vi "PDF Pfad Warnung.vi"(10 "Sprachliste":string[][](array[string]), 11 "String":string) -> ()   [LabVIEW 2015, in "Linearisierung.lvlib"]
uses:
  Linearisierung/Linearisierung.lvlib
  Sprachverwaltung/Sprachverwaltung.lvlib
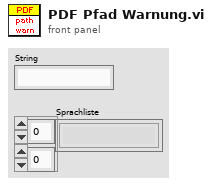
[diagram p1: front panel]
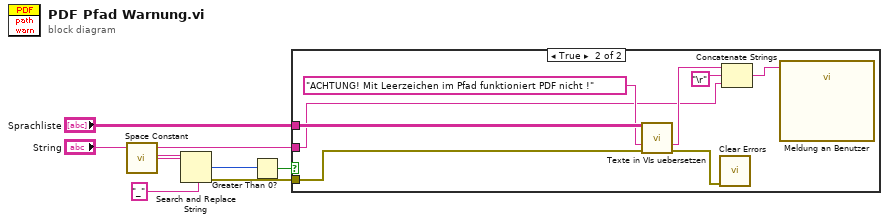
[diagram p0: block diagram]
diagram:
  n1 = call <vilib>:"Space Constant.vi"() -> ("String"=w2:string)
  n2 = Search and Replace String(input string="String", search string=w2, replace string="_") -> (number of replacements=w4:i32, error out=w7:errorcluster)  [unwired: 5 in, 2 out]
  n3 = Greater Than 0?(x=w4) -> (x > 0?=w5:bool)
  n4 = case shown="True" w5 {
    tunnel: "Sprachliste" -> [_ w15]
    tunnel: w7 -> [_ w11]
    tunnel: "String" -> [_ w8]
    frame False {
    }
    frame True {
      n5 = call "Texte in VIs uebersetzen.vi"("Sprachliste"=w15, "String zum Übersetzen"="ACHTUNG! Mit Leerzeichen im Pfad funktioniert PDF nicht !", "error in (no error)"=w11) -> ("String zum Übersetzen"=w13:string, "error out"=w12:errorcluster)  [unwired: 9 in, 2 out]
      n6 = call <vilib>:"Clear Errors.vi"("error in (no error)"=w12) -> ()  [unwired: 5 in, 2 out]
      n7 = Concatenate Strings(w13, "\r", w8) -> (w10:string)
      n8 = call "Meldung an Benutzer"("Message"=w10) -> ()  [unwired: 9 in, 2 out]
    }
  }
